vi "Auto_send_to_MCU.vi"(2 "Message Form":T1, 3 "Types of Data":T2, 4 "MCU Name":string) -> (0 "Send/notsend":bool, 1 "Converted Message":string)   [LabVIEW 2016]
uses:
  Typedef/Type_of_message_to_MCU.ctl
  Typedef/Message_info.ctl
panel:
  out "Byte array has been sent":u8[](array[numeric])
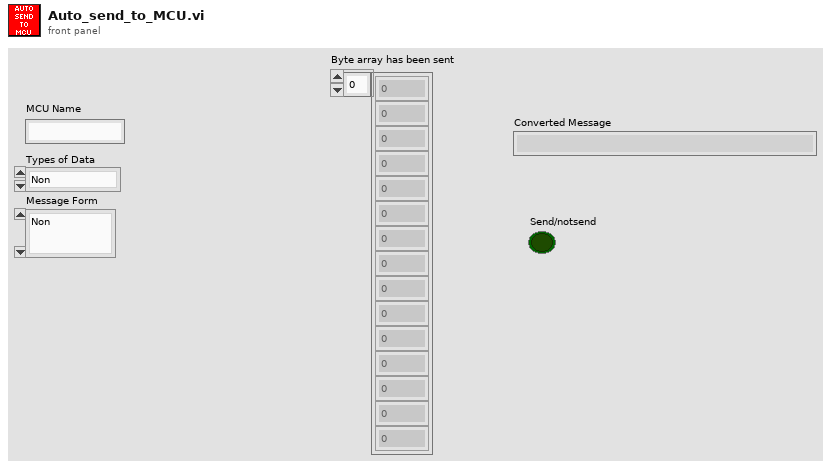
[diagram p1: front panel]
types:
  T1 = typedef "Message_info.ctl" = enum16{"Non", "Earthquake", "Fire", "Lost Power", "New", "Restarted"}
  T2 = typedef "Type_of_message_to_MCU.ctl" = enum16{"Non", "Alarm", "Error", "Time and Date", "Status", "Request"}
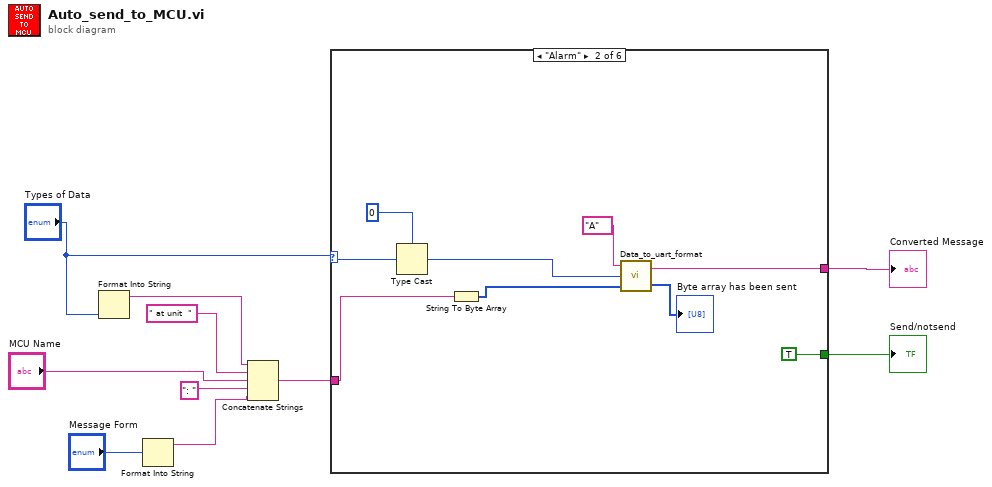
[diagram p0: block diagram]
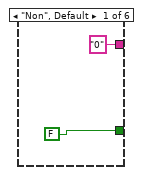
[diagram p2: hidden frame]
diagram:
  n1 = Format Into String("Types of Data") -> (resulting string=w8:string)  [unwired: 3 in, 1 out]
  n2 = Format Into String("Message Form") -> (resulting string=w5:string)  [unwired: 3 in, 1 out]
  n3 = Concatenate Strings(w8, " at unit  " ("string"), "MCU Name", ": " ("string"), w5) -> (w3:string)
  n4 = case shown="\"Alarm\"" "Types of Data" {
    selector: "Types of Data" -> [_ w21 _ _ _ _]
    tunnel: w3 -> [_ w17 _ _ _ _]
    tunnel: [FALSE TRUE _ _ _ _] -> w2
    tunnel: ["0" ("Converted Message") w15 _ _ _ _] -> w1
    frame "Non", Default {
    }
    frame "Alarm" {
      n5 = Type Cast(type=i16 0, x=w21) -> (*(type *) &x=w19:i16)
      n6 = String To Byte Array(string=w17) -> (unsigned byte array=w18:u8[])
      n7 = call "Data_to_uart_format.vi"("Payload  Byte to be sent"=w18, "Types of Data"=w19, "MCU Address to be sent"="A") -> ("Byte array has been sent"=→"Byte array has been sent":u8[], "Converted Message"=w15:string)
    }
    frame "Error" {
    }
    frame "Time and Date" {
    }
    frame "Status" {
    }
    frame "Request" {
    }
  }
  "Send/notsend" <- w2
  "Converted Message" <- w1
